vi "StateScalarStateColorStateName.vi"() -> ()   [LabVIEW 2009]
uses:
  tango_lv8/tango_vi.llb/ReadStateScalarAttribute.vi
panel:
  out "State Name":string
  out "State Color":u32(colorbox)=16448250
  out "error stack":string[](array[string])
  out "State Code":u8
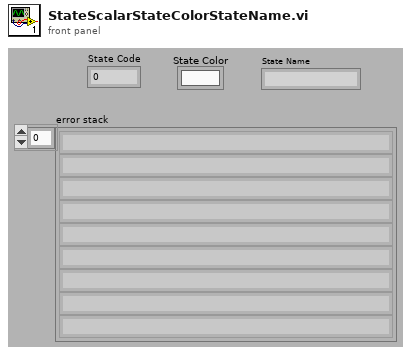
[diagram p1: front panel]
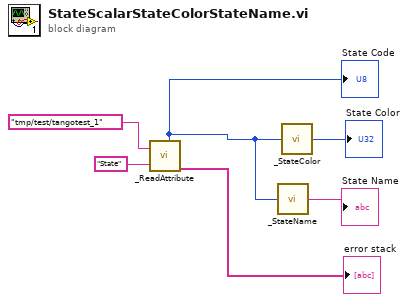
[diagram p0: block diagram]
diagram:
  n1 = call-poly "_ReadAttribute.vi"("device name"="tmp/test/tangotest_1", "attribute name"="State") -> ("value"=w1:i32, "error stack"=→"error stack":string[])  [unwired: 4 out]
  "State Code" <- w1
  n2 = call "_StateName.vi"("State"=w1) -> ("State Name"=→"State Name":string)
  n3 = call "_StateColor.vi"("State"=w1) -> ("State Color"=→"State Color":u32)
